vi "NC_findvar.vi"(3 "name":string, 5 "NC_vararray":T1(array[cluster])) -> (0 "varid":i32, 1 "NC_var":T2, 2 "NC_vararray  out":T1(array[cluster]))   [LabVIEW 2016]
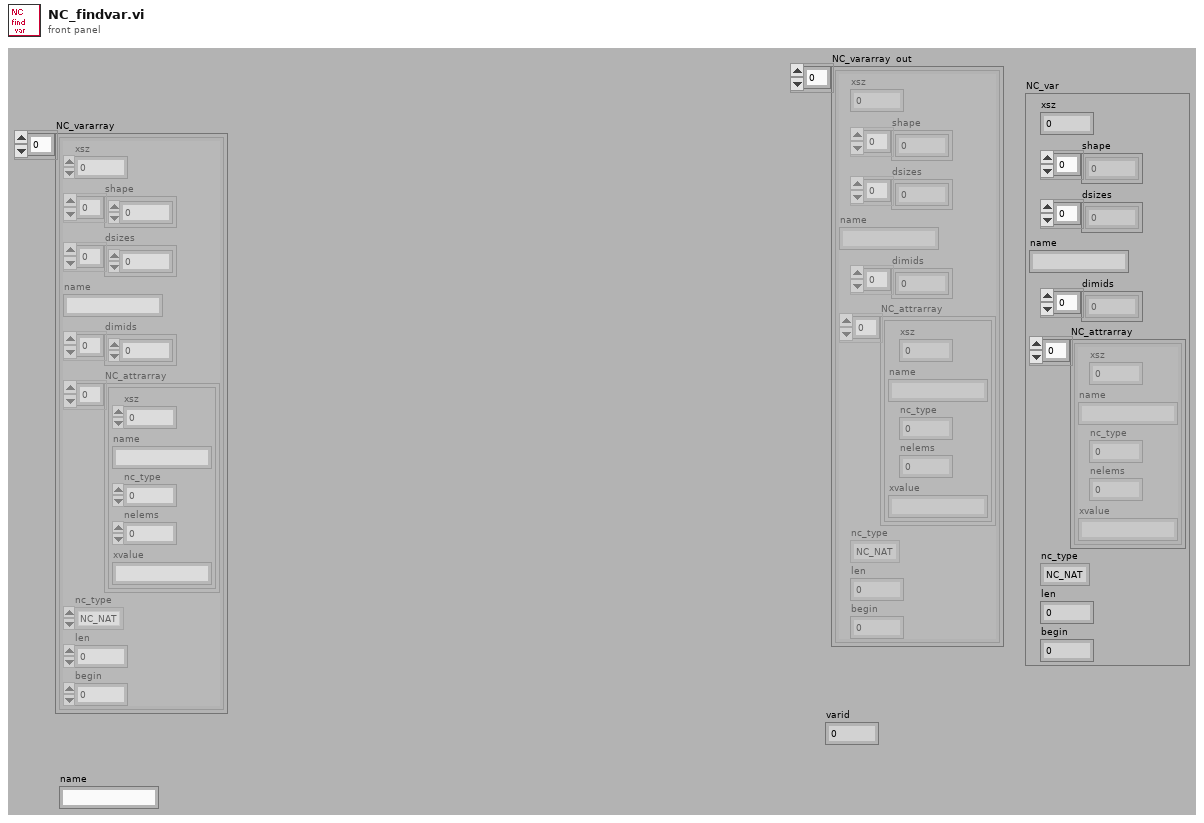
[diagram p1: front panel]
types:
  T1 = cluster{"xsz":u64, "shape":u64[], "dsizes":u64[], "name":string, "dimids":u64[], "NC_attrarray":cluster{"xsz":u64, "name":string, "nc_type":u16, "nelems":u64, "xvalue":string}[], "nc_type":enum16{"NC_NAT", "NC_BYTE", "NC_CHAR", "NC_SHORT", "NC_INT", "NC_FLOAT", "NC_DOUBLE"}, "len":u64, "begin":u64}[]
  T2 = cluster{"xsz":u64, "shape":u64[], "dsizes":u64[], "name":string, "dimids":u64[], "NC_attrarray":cluster{"xsz":u64, "name":string, "nc_type":u16, "nelems":u64, "xvalue":string}[], "nc_type":enum16{"NC_NAT", "NC_BYTE", "NC_CHAR", "NC_SHORT", "NC_INT", "NC_FLOAT", "NC_DOUBLE"}, "len":u64, "begin":u64}
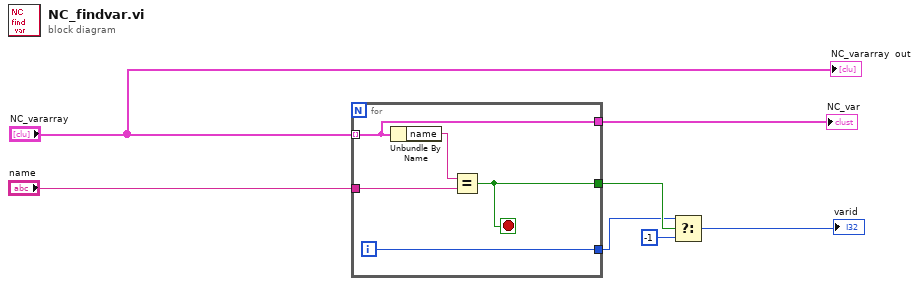
[diagram p0: block diagram]
diagram:
  n1 = for {
    tunnel: "NC_vararray" -> [w8] mode=indexing
    tunnel: "name" -> [w11]
    tunnel: [w10] -> w5
    tunnel: [w9] -> w4
    tunnel: [w8] -> w1
    i -> [w9]
    stop <- w10 stop-if-true
    n2 = Unbundle By Name(w8) -> ("name"=w12:string)
    n3 = Equal?(x=w12, y=w11) -> (x = y?=w10:bool)
  }
  "NC_var" <- w1
  n4 = Select(t=w4, s=w5, f=-1) -> (s? t:f=→"varid":i32)
  "NC_vararray  out" <- "NC_vararray"
